vi "extractModuleName.vi"(8 "error in (no error)":errorcluster, 11 "IDLFile in":refnum<class "IDLFile.lvclass">) -> (0 "error out":errorcluster, 2 "moduleName":string, 3 "IDLFile out":refnum<class "IDLFile.lvclass">)   [LabVIEW 2013, in "IDLFile.lvclass"]
uses:
  IDLFile.lvclass
  IDLFile.lvclass/IDLFile.ctl
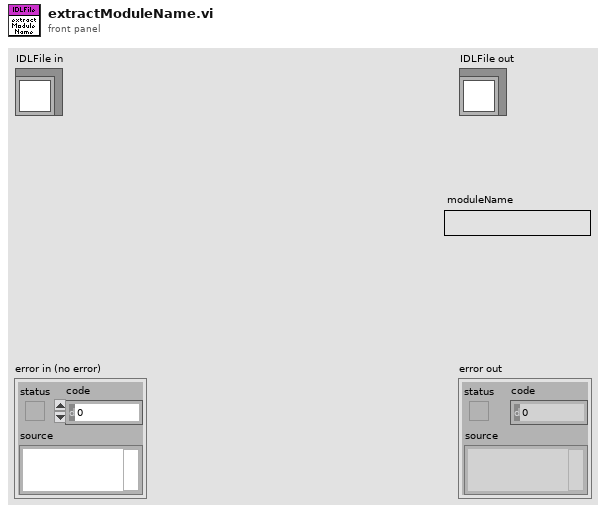
[diagram p1: front panel]
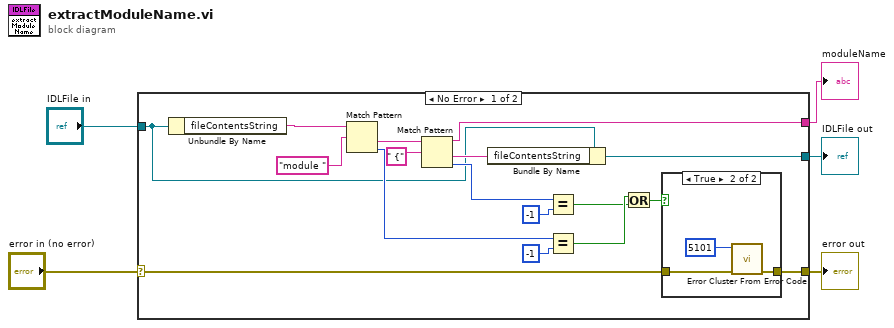
[diagram p0: block diagram]
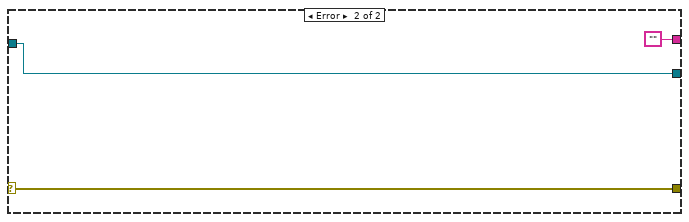
[diagram p3: hidden frame]
diagram:
  n1 = case shown="No Error" "error in (no error)" {
    selector: "error in (no error)" -> [w8 w29]
    tunnel: [w7 w29] -> w4
    tunnel: [w10 w28] -> w2
    tunnel: "IDLFile in" -> [w11 w28]
    tunnel: [w6 ""] -> w1
    frame No Error {
      n2 = Unbundle By Name(w11) -> ("fileContentsString"=w13:string)
      n3 = Match Pattern(string=w13, regular expression="module ") -> (after substring=w21:string, offset past match=w19:i32)  [unwired: 1 in, 2 out]
      n4 = Match Pattern(string=w21, regular expression=" {") -> (before substring=w6:string, after substring=w12:string, offset past match=w17:i32)  [unwired: 1 in, 1 out]
      n5 = Bundle By Name(cluster=w11, "fileContentsString"=w12) -> (w10:refnum<class "IDLFile.lvclass">)
      n6 = Equal?(x=w17, y=-1) -> (x = y?=w14:bool)
      n7 = Equal?(x=w19, y=-1) -> (x = y?=w15:bool)
      n8 = Or(x=w15, y=w14) -> (x .or. y?=w9:bool)
      n9 = case shown="True" w9 {
        tunnel: w8 -> [w23 w25]
        tunnel: [w23 w24] -> w7
        frame False {
        }
        frame True {
          n10 = call <vilib>:"Error Cluster From Error Code.vi"("error in (no error)"=w25, "error code (0)"=5101) -> ("error out"=w24:errorcluster)  [unwired: 7 in]
        }
      }
    }
    frame Error {
    }
  }
  "error out" <- w4
  "IDLFile out" <- w2
  "moduleName" <- w1
